vi "draw_boat_trace.vi"(4 "Radius (px)":dbl=5.0, 6 "circle color":u32(colorbox)=16777215, 8 "Merge Overlay?":bool, 9 "Position":cluster{"X":i32, "Y":i32}, 11 "Image In":T1) -> (3 "Image Out":T1)   [LabVIEW 2013]
doc: "Places a dot on the map showing where the boat has been.\n\n4/5/2014\nMac-I Crowell"
uses:
  <vilib>/vision/Image Controls.llb/IMAQ Image.ctl
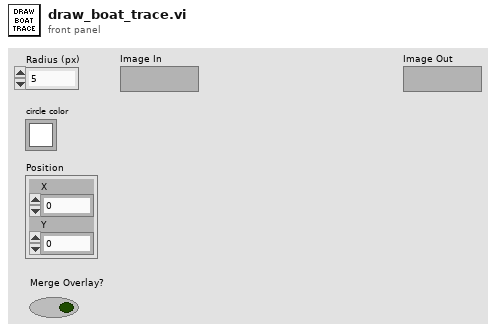
[diagram p1: front panel]
types:
  T1 = typedef "IMAQ Image.ctl" = refnum<image>
  T2 = cluster{"Left":i32, "Top":i32, "Right":i32, "Bottom":i32}
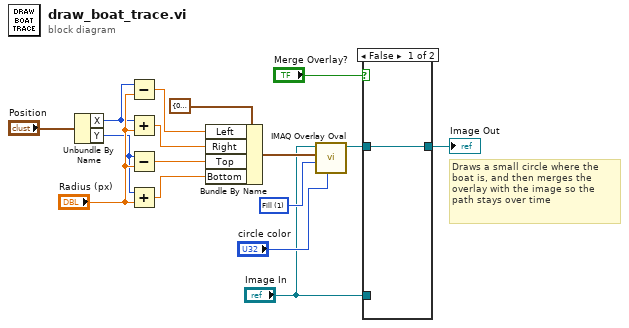
[diagram p0: block diagram]
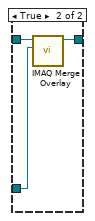
[diagram p2: hidden frame]
diagram:
  w7 = u32 1 items=["Frame", "Fill"] ("Drawing Mode (Frame)")
  # "Draws a small circle where the boat is, and then merges the overlay with the image so the path stays over time"
  n1 = Unbundle By Name("Position") -> ("X"=w13:i32, "Y"=w14:i32)
  n2 = Subtract(x=w13, y="Radius (px)") -> (x-y=w10:dbl)
  n3 = Add(x=w13, y="Radius (px)") -> (x+y=w9:dbl)
  n4 = Subtract(x=w14, y="Radius (px)") -> (x-y=w12:dbl)
  n5 = Add(x=w14, y="Radius (px)") -> (x+y=w11:dbl)
  n6 = Bundle By Name(cluster=T2 {"Left"=0, "Top"=0, "Right"=0, "Bottom"=0} ("Bounding Rectangle"), "Left"=w10, "Right"=w9, "Top"=w12, "Bottom"=w11) -> (w16:T2)
  n7 = call "IMAQ Overlay Oval"("Color"="circle color", "Drawing Mode (Frame)"=w7, "Bounding Rectangle"=w16, "Image"="Image In") -> ("Image Out"=w3:T1)  [unwired: 6 in, 1 out]
  n8 = case shown="False" "Merge Overlay?" {
    tunnel: "Image In" -> [_ w20]
    tunnel: w3 -> [w17 w19]
    tunnel: [w17 w18] -> w2
    frame False {
    }
    frame True {
      n9 = call "IMAQ Merge Overlay"("Image Dst"=w20, "Image Src"=w19) -> ("Image Dst Out"=w18:T1)  [unwired: 8 in, 1 out]
    }
  }
  "Image Out" <- w2
